vi "Format Timestamp.vi"(10 "Time Stamp":timestamp) -> (2 "String":string)   [LabVIEW 2017, in "Cobertura.lvlib"]
uses:
  Cobertura.lvlib
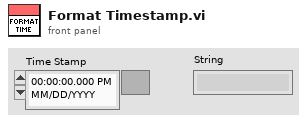
[diagram p1: front panel]
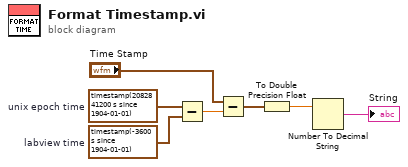
[diagram p0: block diagram]
diagram:
  w6 = timestamp(-3600 s since 1904-01-01)  # labview time
  w7 = timestamp(2082841200 s since 1904-01-01)  # unix epoch time
  n1 = Subtract(x=w7, y=w6) -> (x-y=w5:dbl)
  n2 = Subtract(x="Time Stamp", y=w5) -> (x-y=w2:timestamp)
  n3 = To Double Precision Float(number=w2) -> (double precision float=w1:dbl)
  n4 = Number To Decimal String(number=w1) -> (decimal integer string=→"String":string)  [unwired: 1 in]
